vi "DMM SCOPE 18.vi"() -> ()   [LabVIEW 2021]
uses:
  controls/NaL Ctl 18.ctl
panel:
  in  "Cluster":T1
  in  "Maximum Record Length":dbl=250000000.0 format="%#_6e"
  in  "Sample Rate":dbl=3125000000.0
  out "Division Number":i32
  in  "Tektronix Scope":refnum<visa-resource-name>
  in  "Load DMM Measurement":T2(ring) caption="SMU DMM Measurement"
  in  "Load DMM":refnum<k15>="Dev1"
  out "Load Voltage":dbl caption="SMU Measurement" format="%.6p"
  in  "SMU Resolution in Digits":dbl(ring)=5.5 items=["3 1/2"=3.5, "4 1/2"=4.5, "5 1/2"=5.5, "6 1/2"=6.5, "7 1/2"=7.5]
  in  "SMU DMM Measurement":T2(ring)
  in  "SMU DMM":refnum<k15>="Dev1"
  out "SMU Measurement":dbl format="%.6p"
  in  "error in":errorcluster
  out "error out":errorcluster
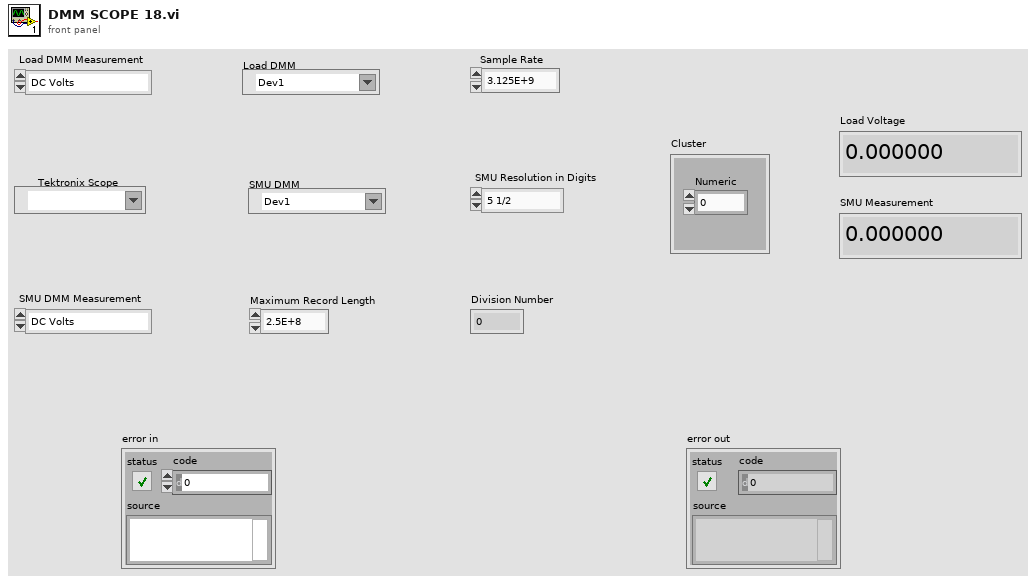
[diagram p1: front panel]
types:
  T1 = typedef "NaL Ctl 18.ctl" = cluster{"Numeric":dbl}
  T2 = enum16{"DC Volts", "AC Volts", "DC Current", "AC Current", "2-wire Resistance", "4-wire Resistance", "Diode", "Frequency", "Period", "AC Volts DC Coupled", "Capacitance", "Inductance", "Temperature"}
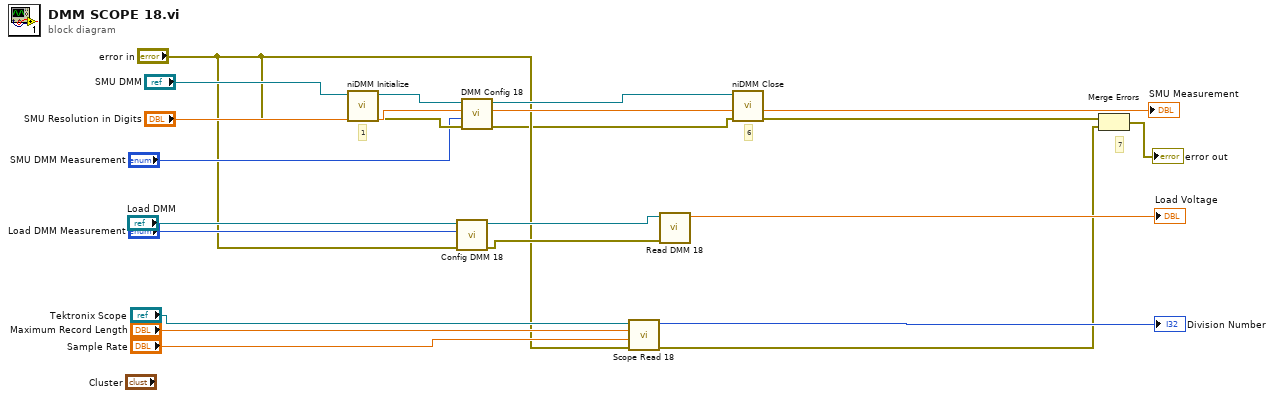
[diagram p0: block diagram]
diagram:
  # "1"
  # "7"
  # "6"
  n1 = call <instrlib>:"niDMM Initialize.vi"("error in (no error)"="error in", "Instrument Descriptor"="SMU DMM") -> ("error out"=w12:errorcluster, "instrument handle out"=w13:refnum<k15>)  [unwired: 8 in]
  n2 = call "Config DMM 18.vi"("error in (no error)"="error in", "Load DMM Measurement"="Load DMM Measurement", "IVI Refnum in"="Load DMM") -> ("error out"=w19:errorcluster, "IVI Refnum out"=w18:refnum<k15>)  [unwired: 7 in]
  n3 = call "DMM Config 18.vi"("error in (no error)"=w12, "SMU DMM Measurement"="SMU DMM Measurement", "SMU Resolution in Digits"="SMU Resolution in Digits", "IVI Refnum in"=w13) -> ("error out"=w1:errorcluster, "Measurement"=→"SMU Measurement":dbl, "IVI Refnum out"=w14:refnum<k15>)  [unwired: 5 in]
  n4 = call "Scope Read 18.vi"("error in (no error)"="error in", "Sample Rate"="Sample Rate", "Maximum Record Length"="Maximum Record Length", "VISA Refnum in"="Tektronix Scope") -> ("error out"=w2:errorcluster, "Division Number"=→"Division Number":i32)  [unwired: 6 in]
  n5 = call "Read DMM 18.vi"("error in (no error)"=w19, "IVI Refnum in"=w18) -> ("Measurement"=→"Load Voltage":dbl)  [unwired: 9 in]
  n6 = call <instrlib>:"niDMM Close.vi"("error in (no error)"=w1, "instrument handle"=w14) -> ("error out"=w8:errorcluster)  [unwired: 9 in]
  n7 = Merge Errors(w8, w2) -> (→"error out":errorcluster)
